vi "FTW-ActorConfig-FormatInitTimeout.vi"(0 "FTW Config String In":string="{}", 7 "Init Timeout":i32=-2, 11 "error in":errorcluster) -> (4 "FTW Config String":string, 15 "error out":errorcluster)   [LabVIEW 2015]
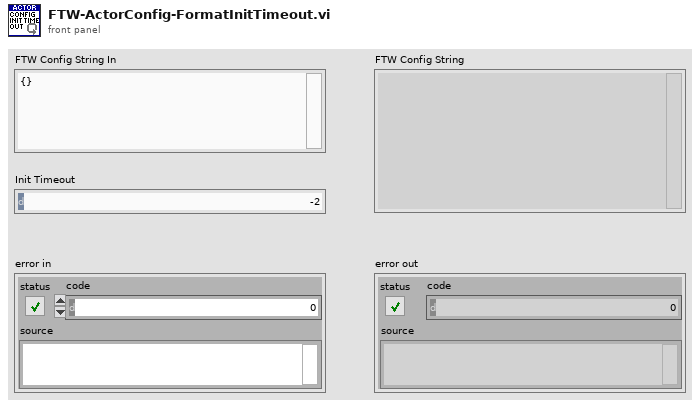
[diagram p1: front panel]
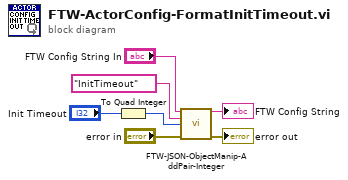
[diagram p0: block diagram]
diagram:
  n1 = To Quad Integer(1:"Init Timeout") -> (0:w4:i64)
  n2 = call "FTW-JSON-ObjectManip-AddPair-Integer.vi"("Input JSON Object"="FTW Config String In", "Key"="InitTimeout", "Value"=w4, "error in"="error in") -> ("Output JSON Object"=→"FTW Config String":string, "error out"=→"error out":errorcluster)  [unwired: 10 in]
